vi "Set Up Dialog - Polar Heart Rate.vi"() -> ()   [LabVIEW 2012]
panel:
  in  "Done":bool
  # "iWorx - Polar Heart Rate - Set Up"
  # "Calibration Instructions"
  # "1. Use warm water to moisten the contact surface of the heart rate belt, then wrap it snuggly directly on the skin around the chest.\n\n2. Snap the Polar heart sensor to the belt; make sure both snaps are connected.\n\n3. Connect the IX-MYDAQ Sensor Adaptor to the NI myDAQ. \n\n4. Connect the PHRMN-100 polar heart rate monitor to the IX-MYDAQ .                                                                                                                                                                          \n5. Connect the NI myDAQ to your computer with a USB cable.\n\n6. Once you see the heart signal on the waveform chart, press the Calibrate button to automatically set the threshold."
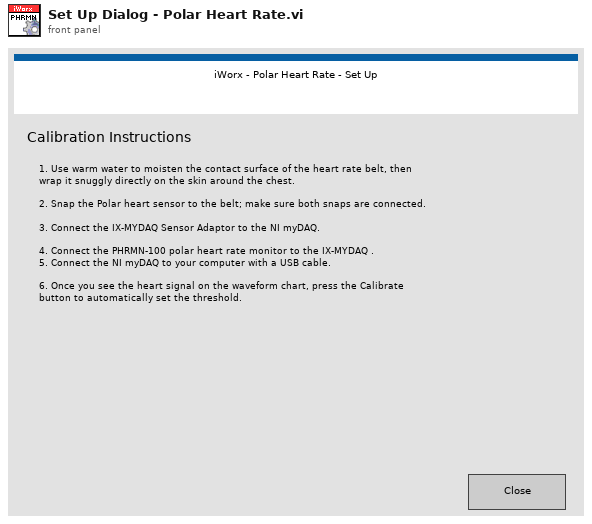
[diagram p1: front panel]
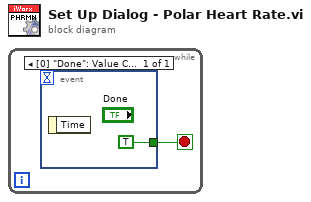
[diagram p0: block diagram]
diagram:
  n1 = while {
    stop <- w1 stop-if-true
    n2 = event shown="[0] \"Done\": Value Change;  Panel Close" {
      selector: _ -> [_]
      dyn-events: _ -> [_]
      timeout: _ -> [_]
      tunnel: [TRUE] -> w1
      event "Done": Value Change; Panel Close {
        n3 = event-data() -> ()  [unwired: 1 in, 1 out]
      }
    }
  }
